vi "Init PowerSupply.vi"(8 "error in (no error)":errorcluster, 11 "BK-Fix-PSU in":refnum<class "BK-Fix-PSU.lvclass">) -> (0 "error out":errorcluster, 3 "BK-Fix-PSU out":refnum<class "BK-Fix-PSU.lvclass">)   [LabVIEW 2020, in "LAF2024Q2.lvlib" / "BK-Fix-PSU.lvclass"]
uses:
  BK-Fix-PSU.lvclass
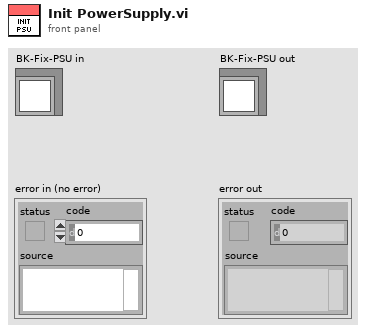
[diagram p1: front panel]
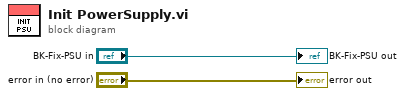
[diagram p0: block diagram]
diagram:
  "error out" <- "error in (no error)"
  "BK-Fix-PSU out" <- "BK-Fix-PSU in"
